vi "DAQmx Create Channel (AI-Torque-Bridge-Two-Point-Linear).vi"(0 "task in":refnum<k21>, 1 "maximum value":dbl=100.0 format="%0.2f", 2 "minimum value":dbl=-100.0 format="%0.2f", 3 "bridge information":T1={"bridge configuration"=10182, "voltage excitation source"=10200, "voltage excitation value"=2.5, "nominal bridge resistance"=350.0} {"voltage excitation source" items=["Internal"=10200, "External"=10167]; "bridge configuration" items=["Full Bridge"=10182, "Half Bridge"=10187, "Quarter Bridge"=10270]}, 5 "physical channels":tag, 7 "name to assign":string, 9 "units":i32(ring)=15883 items=["Nm"=15881, "oz-in"=15882, "lb-in"=15883, "lb-ft"=15884, "From Custom Scale"=10065], 11 "error in":errorcluster, 12 "custom scale name":tag, 14 "scaling information":T2={"first electrical value"=0.0, "second electrical value"=2.0, "electrical units"=15897, "first physical value"=0.0, "second physical value"=100.0, "physical units"=15883} {"physical units" items=["Nm"=15881, "oz-in"=15882, "lb-in"=15883, "lb-ft"=15884]; "electrical units" items=["Volts/Volt"=15896, "mVolts/Volt"=15897]}) -> (4 "task out":refnum<k21>, 15 "error out":errorcluster)   [LabVIEW 2020]
doc: "Creates channel(s) that use a Wheatstone bridge to measure torque. Use this instance with sensors whose specifications do not provide a polynomial for scaling or a table of electrical and physical values. When you use this scaling type, NI-DAQmx uses two points of electrical and physical values to calculate the slope and y-intercept of a linear equation and uses that equation to scale electrical values to physical values."
uses:
  nilvaiu.dll
panel:
  # "input limits"
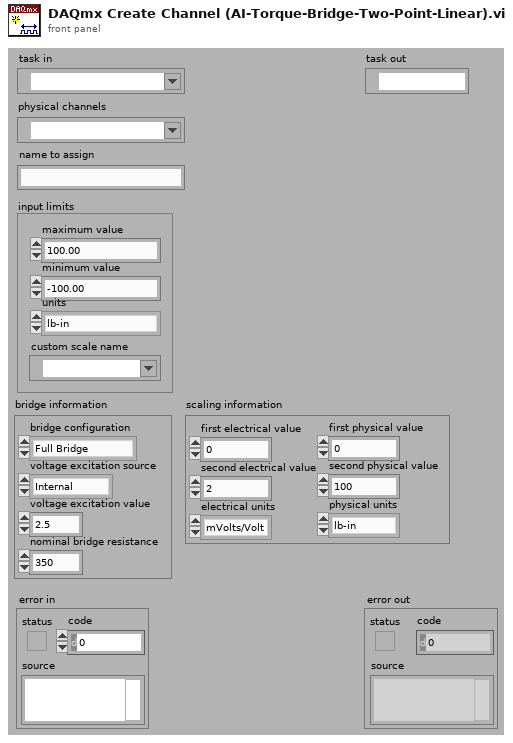
[diagram p1: front panel]
types:
  T1 = cluster{"bridge configuration":i32, "voltage excitation source":i32, "voltage excitation value":dbl, "nominal bridge resistance":dbl}
  T2 = cluster{"first electrical value":dbl, "second electrical value":dbl, "electrical units":i32, "first physical value":dbl, "second physical value":dbl, "physical units":i32}
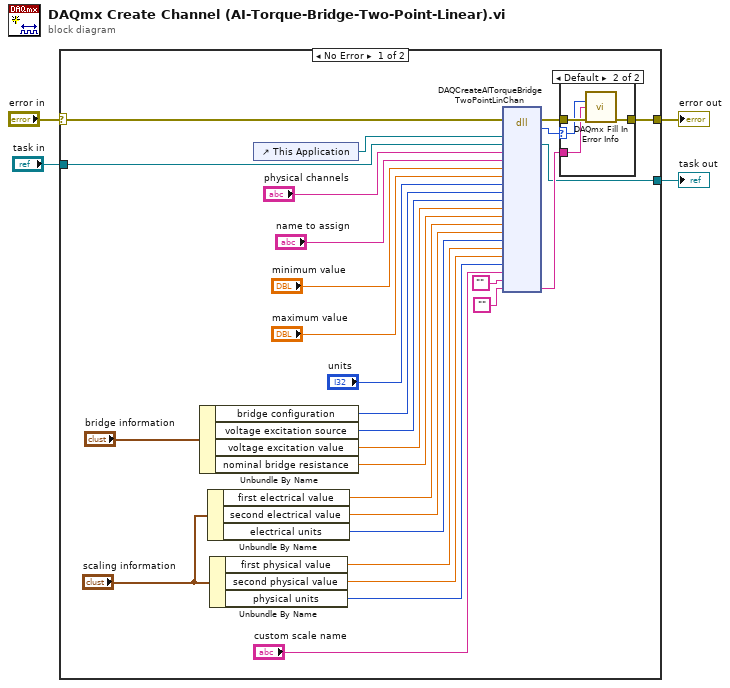
[diagram p0: block diagram]
diagram:
  n1 = case shown="No Error" "error in" {
    selector: "error in" -> [w8 w38]
    tunnel: "task in" -> [w10 w39]
    tunnel: [w9 w39] -> w3
    tunnel: [w7 w38] -> w1
    frame No Error {
      n2 = Unbundle By Name("bridge information") -> ("bridge configuration"=w26:i32, "voltage excitation source"=w27:i32, "voltage excitation value"=w28:dbl, "nominal bridge resistance"=w29:dbl)
      n3 = Unbundle By Name("scaling information") -> ("first electrical value"=w20:dbl, "second electrical value"=w21:dbl, "electrical units"=w22:i32)
      n4 = Unbundle By Name("scaling information") -> ("first physical value"=w23:dbl, "second physical value"=w24:dbl, "physical units"=w25:i32)
      n5 = control-ref of="This Application"() -> (w14:refnum<vi>)
      n6 = dll-call lib="nilvaiu.*" fn="DAQCreateAITorqueBridgeTwoPointLinChan"(error in=w8, "lvAppRef"=w14, "refObjPtr"=w10, "physicalChannelName"="physical channels", "channelNameIn"="name to assign", "minVal"="minimum value", "maxVal"="maximum value", "units"="units", "bridgeConfig"=w26, "voltageExcitSource"=w27, "voltageExcitVal"=w28, "nominalBridgeResistance"=w29, "firstElectricalValue"=w20, "secondElectricalValue"=w21, "electricalUnits"=w22, "firstPhysicalValue"=w23, "secondPhysicalValue"=w24, "physicalUnits"=w25, "customScaleName"="custom scale name", "channelNamesOut"="", "extendedErrorInfo"="") -> (error out=w32:errorcluster, "return type"=w30:i32, "refObjPtr"=w9:refnum<k21>, "extendedErrorInfo"=w31:string)  [unwired: 20 in, 1 out]
      n7 = case shown="Default" w30 {
        selector: w30 -> [_ w35]
        tunnel: w32 -> [w33 w37]
        tunnel: [w33 w36] -> w7
        tunnel: w31 -> [_ w34]
        frame 0 {
        }
        frame Default {
          n8 = call "DAQmx Fill In Error Info.vi"("status code"=w35, "extended error info"=w34, "error in"=w37) -> ("error out"=w36:errorcluster)  [unwired: 1 in, 11 out]
        }
      }
    }
    frame Error {
    }
  }
  "task out" <- w3
  "error out" <- w1
